vi "FPGA_EncoderWriteReset.vi"(8 "error in (no error)":errorcluster, 11 "EncoderDevRef":T1) -> (0 "error out":errorcluster, 3 "EncoderDevRef":T1)   [LabVIEW 2017]
uses:
  <vilib>/Rock Robotics/SystemInterfaces/Encoder/FPGA_EncoderDevRef.ctl
  <vilib>/Rock Robotics/SystemInterfaces/Encoder/FPGA_EncoderIdx.ctl
  <vilib>/Rock Robotics/SystemInterfaces/System/FPGA_SystemFPGA Ref Global.vi
  <vilib>/Utility/error.llb/Error Cluster From Error Code.vi
  <vilib>/rvi/errors/niLvFpgaAdjustHostInterfaceError.vi
  <vilib>/rvi/interface/nirviReadWriteControl/nirviReadWriteControl.xnode
  <vilib>/Rock Robotics/SystemInterfaces/System/FPGA_SystemFRC FPGA Ref.ctl
  NiFpgaLv.dll
  <vilib>/rvi/interface/Simulation/niFpgaSimulationCallBeginRW.vi
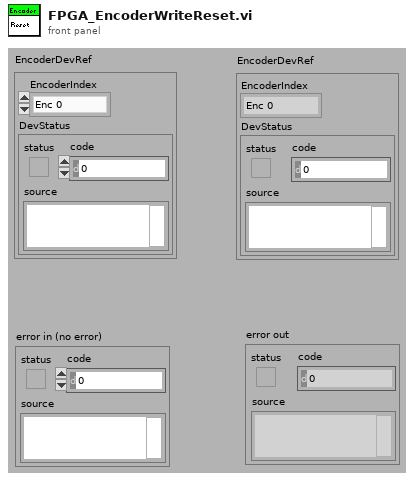
[diagram p1: front panel]
types:
  T1 = typedef "FPGA_EncoderDevRef.ctl" = cluster{"EncoderIndex":T2, "DevStatus":errorcluster}
  T2 = typedef "FPGA_EncoderIdx.ctl" = enum8{"Enc 0", "Enc 1", "Enc 2", "Enc 3", "Enc 4", "Enc 5", "Enc 6", "Enc 7", "Invalid"}
  T3 = typedef "FPGA_SystemFRC FPGA Ref.ctl" = refnum<k20>
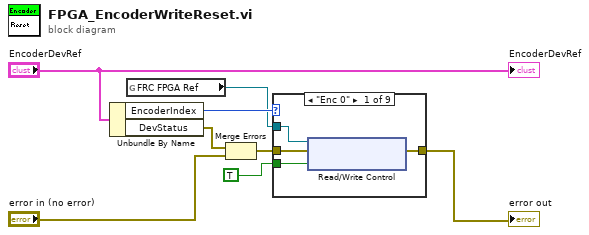
[diagram p0: block diagram]
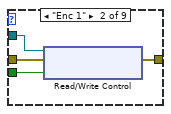
[diagram p2: hidden frame]
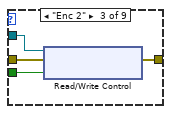
[diagram p3: hidden frame]
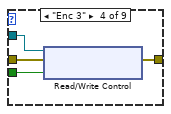
[diagram p4: hidden frame]
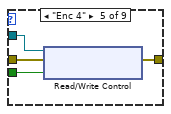
[diagram p5: hidden frame]
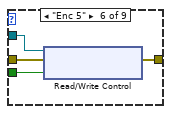
[diagram p6: hidden frame]
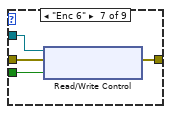
[diagram p7: hidden frame]
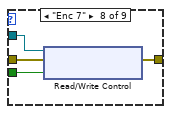
[diagram p8: hidden frame]
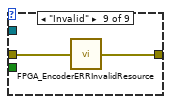
[diagram p9: hidden frame]
diagram:
  n1 = Unbundle By Name("EncoderDevRef") -> ("EncoderIndex"=w6:T2, "DevStatus"=w3:errorcluster)
  n2 = global read "FPGA_SystemFPGA Ref Global.vi" "FRC FPGA Ref"() -> (w4:T3)
  n3 = Merge Errors(w3, "error in (no error)") -> (w2:errorcluster)
  n4 = case shown="\"Enc 0\"" w6 {
    tunnel: w4 -> [w9 w13 w17 w21 w25 w29 w33 w37 _]
    tunnel: w2 -> [w10 w14 w18 w22 w26 w30 w34 w38 w42]
    tunnel: [w11 w15 w19 w23 w27 w31 w35 w39 w41] -> w7
    tunnel: TRUE ("Reset") -> [w12 w16 w20 w24 w28 w32 w36 w40 _]
    frame "Enc 0" {
      n5 = xnode "Read/Write Control"("FPGA VI Reference In"=w9, "error in"=w10, "Encoder0.Reset"=w12) -> ("error out"=w11:errorcluster)  [unwired: 1 out]
    }
    frame "Enc 1" {
      n6 = xnode "Read/Write Control"("FPGA VI Reference In"=w13, "error in"=w14, "Encoder1.Reset"=w16) -> ("error out"=w15:errorcluster)  [unwired: 1 out]
    }
    frame "Enc 2" {
      n7 = xnode "Read/Write Control"("FPGA VI Reference In"=w17, "error in"=w18, "Encoder2.Reset"=w20) -> ("error out"=w19:errorcluster)  [unwired: 1 out]
    }
    frame "Enc 3" {
      n8 = xnode "Read/Write Control"("FPGA VI Reference In"=w21, "error in"=w22, "Encoder3.Reset"=w24) -> ("error out"=w23:errorcluster)  [unwired: 1 out]
    }
    frame "Enc 4" {
      n9 = xnode "Read/Write Control"("FPGA VI Reference In"=w25, "error in"=w26, "Encoder4.Reset"=w28) -> ("error out"=w27:errorcluster)  [unwired: 1 out]
    }
    frame "Enc 5" {
      n10 = xnode "Read/Write Control"("FPGA VI Reference In"=w29, "error in"=w30, "Encoder5.Reset"=w32) -> ("error out"=w31:errorcluster)  [unwired: 1 out]
    }
    frame "Enc 6" {
      n11 = xnode "Read/Write Control"("FPGA VI Reference In"=w33, "error in"=w34, "Encoder6.Reset"=w36) -> ("error out"=w35:errorcluster)  [unwired: 1 out]
    }
    frame "Enc 7" {
      n12 = xnode "Read/Write Control"("FPGA VI Reference In"=w37, "error in"=w38, "Encoder7.Reset"=w40) -> ("error out"=w39:errorcluster)  [unwired: 1 out]
    }
    frame "Invalid" {
      n13 = call <vilib>:"FPGA_EncoderERRInvalidResource.vi"("error in (no error)"=w42) -> ("error out"=w41:errorcluster)
    }
  }
  "error out" <- w7
  "EncoderDevRef" <- "EncoderDevRef"
